vi "Construct New Filename Ver013.vi"(0 "Original Filename":path, 1 "Completely New Filename (uses same PATH)":string, 2 "New Prefix String to add to the Original Filename":string="PARSED_", 3 "New Extension":string="txt") -> (6 "New Filename with Path":path, 7 "New Filename as a STRING":string, 8 "Original Filename as a String":string, 9 "Status (0:OK, -1: Fault)":i32, 10 "Completely New Filename\nwith Same PATH":path)   [LabVIEW 2017]
panel:
  out "Elements of New Filename Path":string[](array[string])
  out "Original Filename Extension (.TXT)":string
  out "Original Filename w/o Prefix":string
  out "Elements of the Original Filename":string[](array[string])
  # "Take the Original Filename (with path) and create a New Filename"
  # "EXAMPLE:  JudyBLUE.txt"
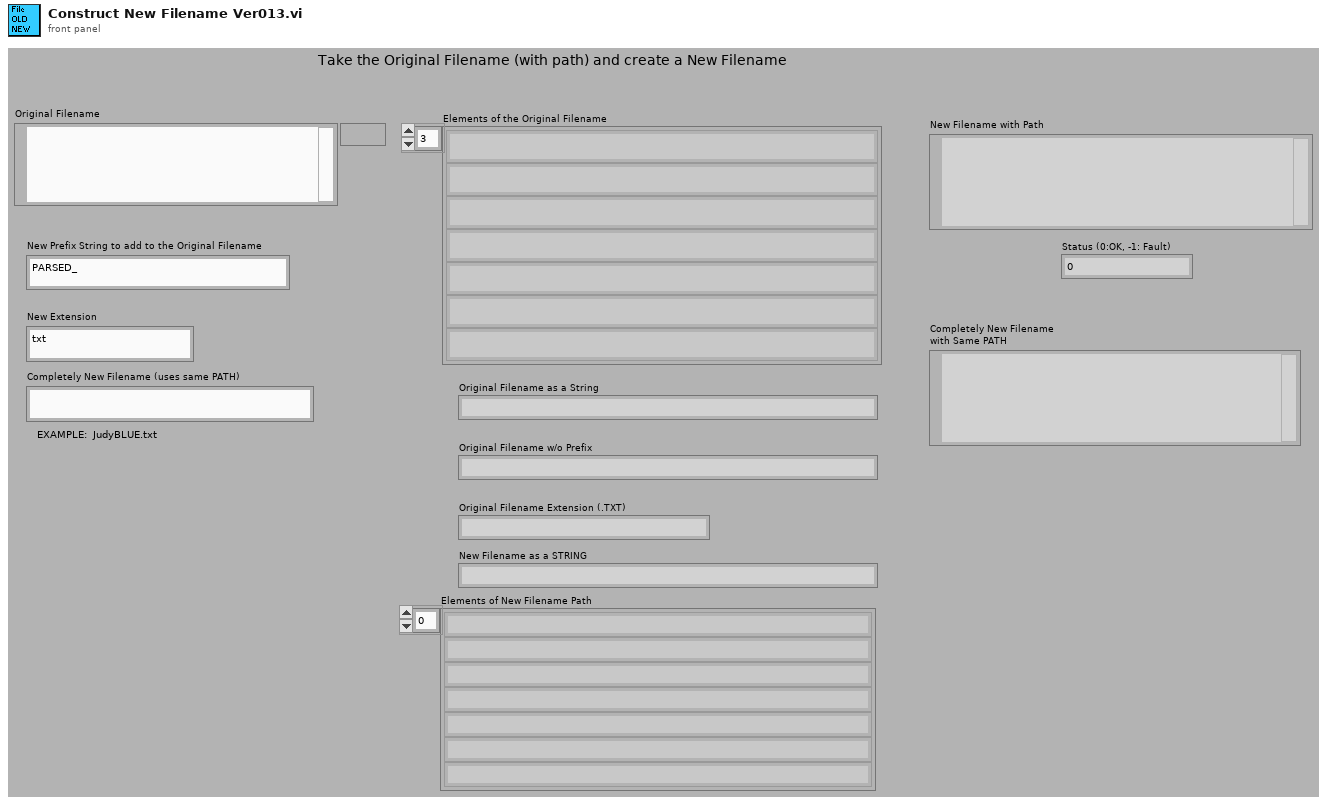
[diagram p1: front panel]
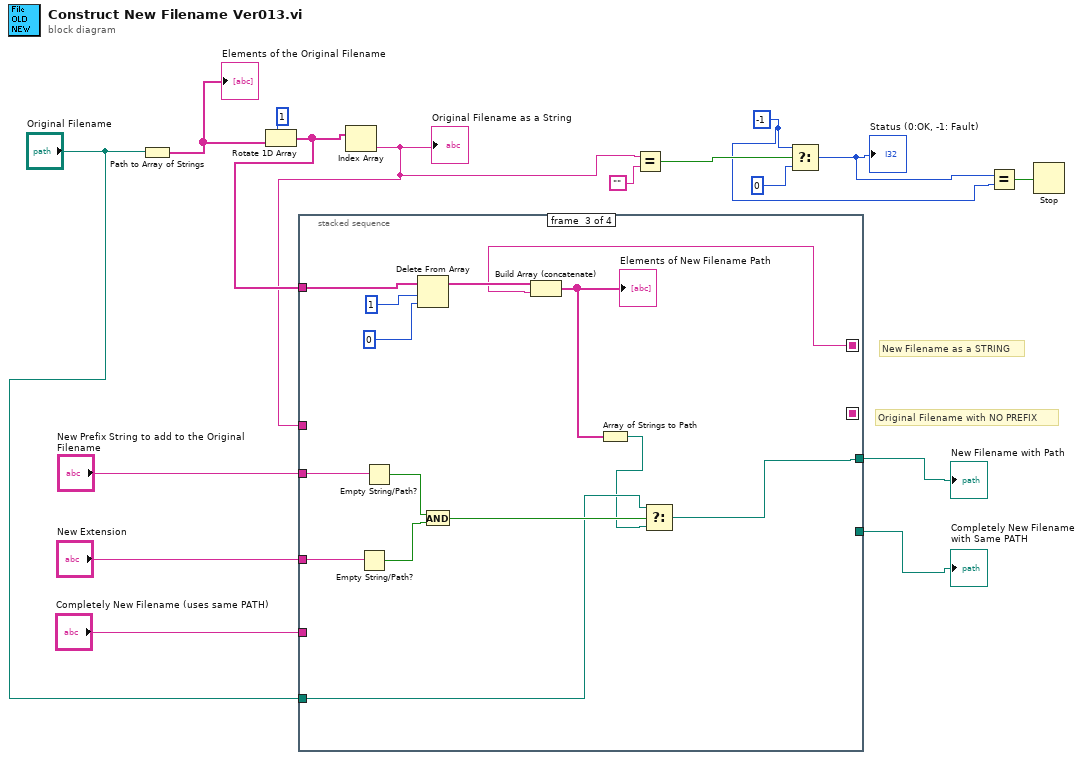
[diagram p0: block diagram]
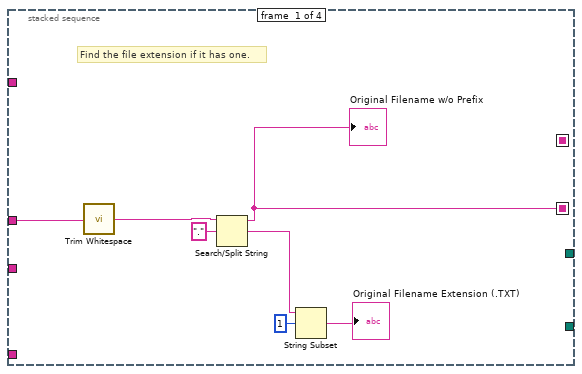
[diagram p2: hidden frame]
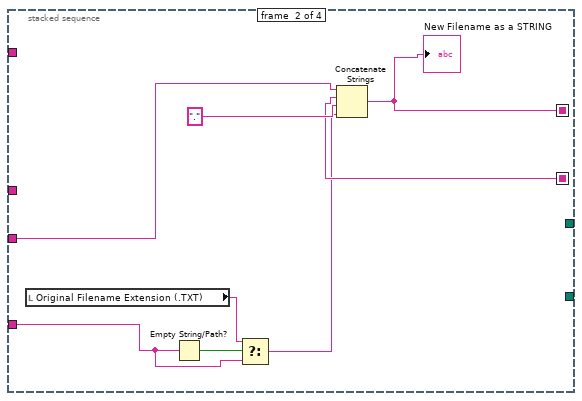
[diagram p3: hidden frame]
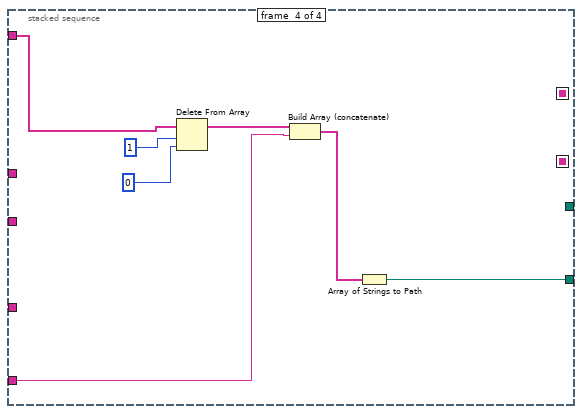
[diagram p4: hidden frame]
diagram:
  w5 = -1
  # "New Filename as a STRING"
  # "Original Filename with NO PREFIX"
  n1 = Path to Array of Strings(0:"Original Filename") -> (2:w16:string[])  [unwired: 1 out]
  "Elements of the Original Filename" <- w16
  n2 = Rotate 1D Array(1:w16, 2:1 ("n")) -> (0:w12:string[])
  n3 = Index Array(array=w12) -> (element=w10:string)  [unwired: 1 in]
  "Original Filename as a String" <- w10
  n4 = stacked-sequence {
    seq-local: [w20 _ _ _] -> [_ w29 _ _]
    seq-local: [_ w28 _ _] -> [_ _ w41 _]
    tunnel: w10 -> [w22 _ _ _]
    tunnel: "New Prefix String to add to the Original Filename" -> [_ w31 w39 _]
    tunnel: "New Extension" -> [_ w26 w38 _]
    tunnel: w12 -> [_ _ w45 w48]
    tunnel: [_ _ w32 _] -> w11
    tunnel: "Completely New Filename (uses same PATH)" -> [_ _ _ w47]
    tunnel: [_ _ _ w46] -> w2
    tunnel: "Original Filename" -> [_ _ w34 _]
    frame #0 {
      # "Find the file extension if it has one."
      n5 = call <vilib>:"Trim Whitespace.vi"("string"=w22) -> ("trimmed string"=w21:string)  [unwired: 1 in]
      n6 = Search/Split String(string=w21, search string/char (-)="." ("regular expression")) -> (substring before match=w20:string, match + rest of string=w18:string)  [unwired: 2 out]
      "Original Filename w/o Prefix" <- w20
      n7 = String Subset(string=w18, offset (0)=1) -> (substring=→"Original Filename Extension (.TXT)":string)  [unwired: 1 in]
    }
    frame #1 {
      n8 = local read "Original Filename Extension (.TXT)"() -> (w25:string)
      n9 = Empty String/Path?(string/path=w26) -> (empty?=w27:bool)
      n10 = Select(t=w25, s=w27, f=w26) -> (s? t:f=w24:string)
      n11 = Concatenate Strings(w31, w29, "." ("string"), w24) -> (w28:string)
      "New Filename as a STRING" <- w28
    }
    frame #2 {
      n12 = Empty String/Path?(string/path=w38) -> (empty?=w36:bool)
      n13 = Empty String/Path?(string/path=w39) -> (empty?=w37:bool)
      n14 = Delete From Array(array=w45, length=1, index=0) -> (array with subset deleted=w42:string[])  [unwired: 1 out]
      n15 = And(x=w37, y=w36) -> (x .and. y?=w35:bool)
      n16 = Build Array (concatenate)(w42, w41) -> (w40:string[])
      "Elements of New Filename Path" <- w40
      n17 = Array of Strings to Path(0:w40) -> (2:w33:path)  [unwired: 1 out]
      n18 = Select(t=w34, s=w35, f=w33) -> (s? t:f=w32:path)
    }
    frame #3 {
      n19 = Delete From Array(array=w48, length=1, index=0) -> (array with subset deleted=w50:string[])  [unwired: 1 out]
      n20 = Build Array (concatenate)(w50, w47) -> (w49:string[])
      n21 = Array of Strings to Path(0:w49) -> (2:w46:path)  [unwired: 1 out]
    }
  }
  "New Filename with Path" <- w11
  "Completely New Filename\nwith Same PATH" <- w2
  n22 = Equal?(x=w10, y="") -> (x = y?=w8:bool)
  n23 = Select(t=w5, s=w8, f=0 ("index")) -> (s? t:f=w6:i32)
  "Status (0:OK, -1: Fault)" <- w6
  n24 = Equal?(x=w6, y=w5) -> (x = y?=w4:bool)
  n25 = Stop(stop? (T)=w4) -> ()
